vi "Initialize.vi"(8 "error in (no error)":errorcluster, 11 "CT-De-energizeThenStop-Cmd in":refnum<class "CT-De-energizeThenStop-Cmd.lvclass">) -> (0 "error out":errorcluster, 3 "CT-De-energizeThenStop-Cmd out":refnum<class "CT-De-energizeThenStop-Cmd.lvclass">)   [LabVIEW 2013, in "CT-De-energizeThenStop-Cmd.lvclass"]
uses:
  CT-De-energizeThenStop-Cmd.lvclass
  Systems/GrabberArms/GrabberArms.lvclass
  States/CT-GrabberInWay-State/CT-GrabberInWay-State.lvclass
  States/CT-De-Energizing-State/CT-De-Energizing-State.lvclass
  Robot Global Data.vi
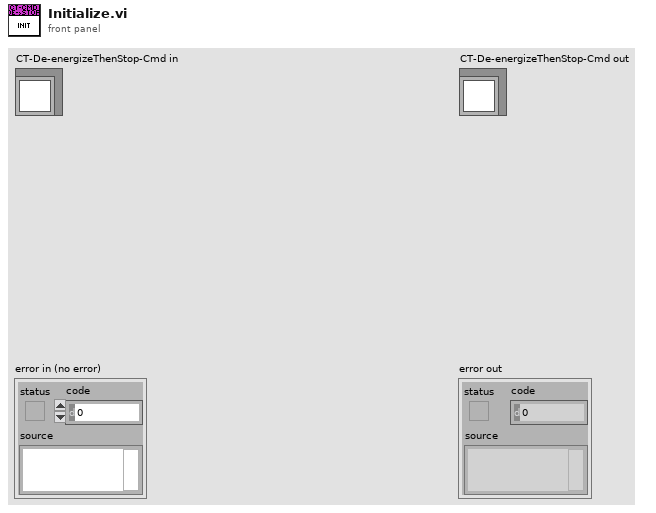
[diagram p1: front panel]
types:
  T1 = typedef "WPI_DigitalInputDevRef.ctl" = cluster{"DevStatus":errorcluster, "DIO Channel":T2, "Digital Module":T3}
  T2 = typedef "FPGA_DIOChannel.ctl" = enum8{"DIO 1", "DIO 2", "DIO 3", "DIO 4", "DIO 5", "DIO 6", "DIO 7", "DIO 8", "DIO 9", "DIO 10", "DIO 11", "DIO 12", "DIO 13", "DIO 14", "Invalid"}
  T3 = typedef "FPGA_TypedefDigitalModule.ctl" = enum16{"Digital Module 1", "Digital Module 2"}
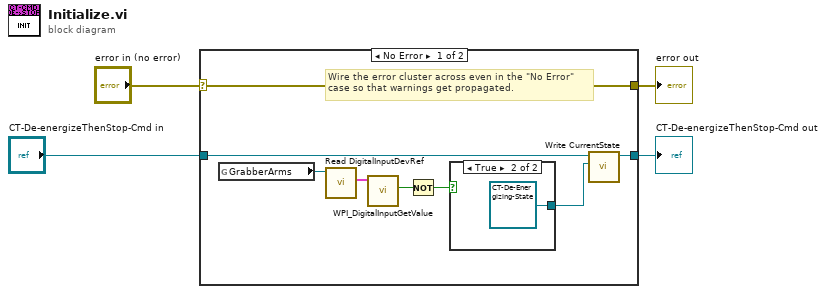
[diagram p0: block diagram]
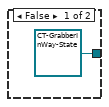
[diagram p2: hidden frame]
diagram:
  n1 = case shown="No Error" "error in (no error)" {
    selector: "error in (no error)" -> [w12 w16]
    tunnel: [w12 w16] -> w3
    tunnel: [w10 w15] -> w1
    tunnel: "CT-De-energizeThenStop-Cmd in" -> [w11 w15]
    frame No Error {
      # "Wire the error cluster across even in the \"No Error\"\ncase so that warnings get propagated."
      n2 = global read "Robot Global Data.vi" "GrabberArms"() -> (w8:refnum<class "GrabberArms.lvclass">)
      n3 = call-dynamic "Read DigitalInputDevRef.vi"("GrabberArms in"=w8) -> ("DigitalInputDevRef"=w7:T1)  [unwired: 8 in, 2 out]
      n4 = call <vilib>:"WPI_DigitalInputGetValue.vi"("DigitalInputDevRef"=w7) -> ("Value"=w6:bool)  [unwired: 8 in, 2 out]
      n5 = Not(x=w6) -> (.not. x?=w5:bool)
      n6 = case shown="True" w5 {
        tunnel: [refnum<class "CT-GrabberInWay-State.lvclass"> refnum ("CT-GrabberInWay-State.lvclass") refnum<class "CT-De-Energizing-State.lvclass"> refnum ("CT-De-Energizing-State.lvclass")] -> w9
        frame False {
        }
        frame True {
        }
      }
      n7 = call-dynamic "Write CurrentState.vi"("State.lvclass"=w9, "Command in"=w11) -> ("Command out"=w10:refnum<class "CT-De-energizeThenStop-Cmd.lvclass">)  [unwired: 8 in, 1 out]
    }
    frame Error {
    }
  }
  "error out" <- w3
  "CT-De-energizeThenStop-Cmd out" <- w1
